vi "InitFPGA.vi"(2 "error in":errorcluster, 3 "FPGA VI In":refnum<k20>) -> (0 "error out":errorcluster, 1 "FPGA VI Reference Out":refnum<k20>)   [LabVIEW 2014]
doc: "Check for compatibility and Initilize FPGA."
uses:
  <vilib>/LabVIEW Targets/FPGA/FlexRIO/CustomFPGAMethods/79XXR_Method_IOModuleStatusImpl.vi
  <vilib>/Utility/error.llb/Error Cluster From Error Code.vi
  <vilib>/rvi/errors/niLvFpgaAdjustHostInterfaceError.vi
  <vilib>/rvi/interface/nirviMethod/nirviMethod.xnode
  <vilib>/rvi/interface/nirviReadWriteControl/nirviReadWriteControl.xnode
  NiFpgaLv.dll
  <vilib>/rvi/interface/Simulation/niFpgaSimulationCallBeginRW.vi
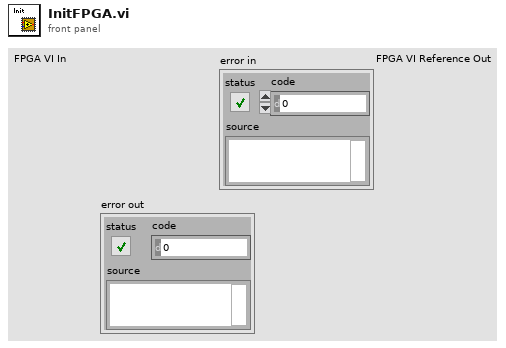
[diagram p1: front panel]
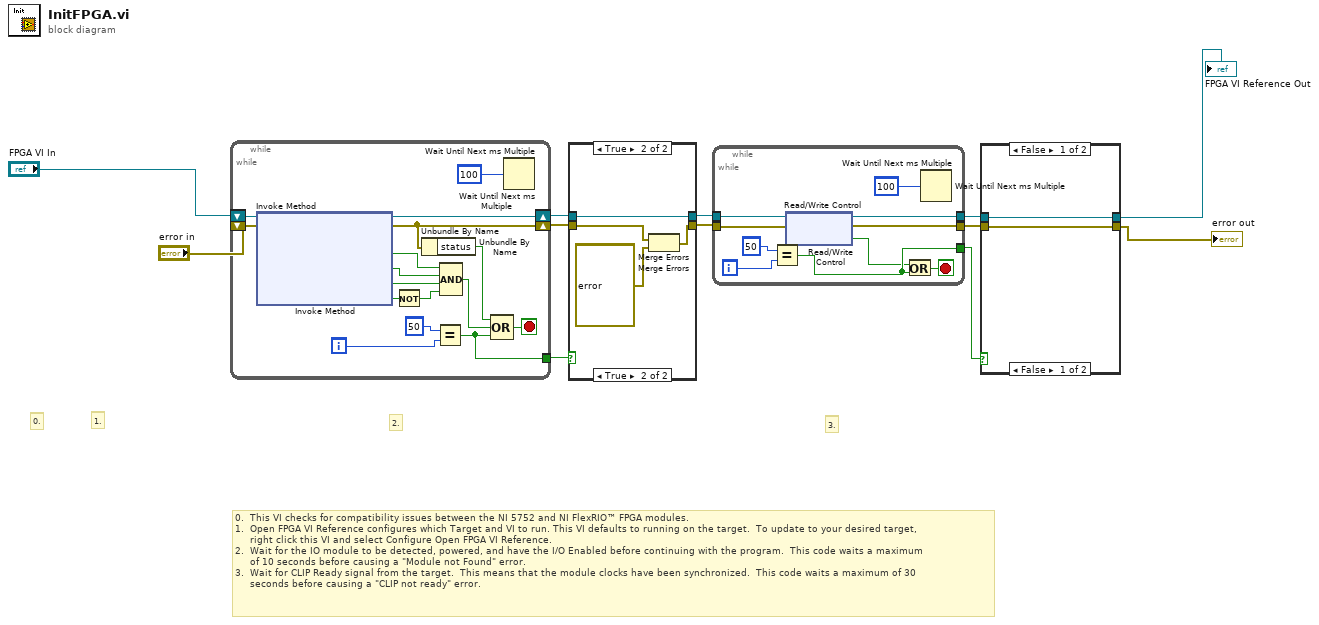
[diagram p0: block diagram]
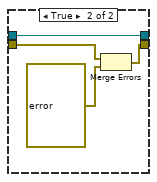
[diagram p2: hidden frame]
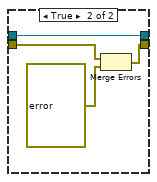
[diagram p4: hidden frame]
diagram:
  # "0.  This VI checks for compatibility issues between the NI 5752 and NI FlexRIO™ FPGA modules. \n1.  Open FPGA VI Reference configures which Target and VI to run. This VI defaults to running on the target.  To update to your desired target, \n     right click this VI and select Configure Open FPGA VI Reference.\n2.  Wait for the IO module to be detected, powered, and have the I/O Enabled before continuing with the program.  This code waits a maximum \n     of 10 seconds before causing a \"Module not Found\" error.\n3.  Wait for CLIP Ready signal from the target.  This means that the module clocks have been synchronized.  This code waits a maximum of 30 \n     seconds before causing a \"CLIP not ready\" error."
  # "0."
  # "3."
  # "1."
  # "0."
  # "3."
  # "2."
  # "1."
  n1 = while {
    shift-right: [w27] -> w20
    shift-left: "error in" -> [w35]
    shift-right: [w34] -> w18
    shift-left: "FPGA VI In" -> [w36]
    tunnel: [w23] -> w19
    i -> [w29]
    stop <- w24 stop-if-true
    n2 = xnode "Invoke Method"("FPGA VI Reference In"=w36, "error in"=w35) -> ("FPGA VI Reference Out"=w34:refnum<k20>, "error out"=w27:errorcluster, "IO Module Present?"=w33:bool, "Power Enabled?"=w32:bool, "IO Enabled?"=w31:bool, "IO Module Mismatch?"=w22:bool)
    n3 = Not(x=w22) -> (.not. x?=w21:bool)
    n4 = Unbundle By Name(w27) -> ("status"=w26:bool)
    n5 = Equal?(x=50, y=w29) -> (x = y?=w23:bool)
    n6 = Compound Arithmetic op=AND(w33, w32, w31, w21) -> (w25:bool)
    n7 = Compound Arithmetic op=OR(w26, w25, w23) -> (w24:bool)
    n8 = Wait Until Next ms Multiple(millisecond multiple=u32 100) -> ()  [unwired: 1 out]
  }
  n9 = while {
    shift-right: [w43] -> w4
    shift-left: _ -> [w51]
    shift-right: [w50] -> w6
    shift-left: _ -> [w52]
    tunnel: [w39] -> w5
    i -> [w45]
    stop <- w40 stop-if-true
    n10 = xnode "Invoke Method"("FPGA VI Reference In"=w52, "error in"=w51) -> ("FPGA VI Reference Out"=w50:refnum<k20>, "error out"=w43:errorcluster, "IO Module Present?"=w49:bool, "Power Enabled?"=w48:bool, "IO Enabled?"=w47:bool, "IO Module Mismatch?"=w38:bool)
    n11 = Not(x=w38) -> (.not. x?=w37:bool)
    n12 = Unbundle By Name(w43) -> ("status"=w42:bool)
    n13 = Equal?(x=50, y=w45) -> (x = y?=w39:bool)
    n14 = Compound Arithmetic op=AND(w49, w48, w47, w37) -> (w41:bool)
    n15 = Compound Arithmetic op=OR(w42, w41, w39) -> (w40:bool)
    n16 = Wait Until Next ms Multiple(millisecond multiple=u32 100) -> ()  [unwired: 1 out]
  }
  n17 = case shown="True" w19 {
    tunnel: w20 -> [w53 w57]
    tunnel: [w53 w56] -> w16
    tunnel: w18 -> [w54 w55]
    tunnel: [w54 w55] -> w17
    frame False {
    }
    frame True {
      n18 = Merge Errors(w57, errorcluster {"status"=TRUE, "code"=-1, "source"="The IO Module was not present, powered, or the IO were not enabled.  Verify the NI 5752 is securly connected and try again."} ("error in")) -> (w56:errorcluster)
    }
  }
  n19 = case shown="True" w5 {
    tunnel: w4 -> [w59 w63]
    tunnel: [w59 w62] -> w8
    tunnel: w6 -> [w60 w61]
    tunnel: [w60 w61] -> w7
    frame False {
    }
    frame True {
      n20 = Merge Errors(w63, errorcluster {"status"=TRUE, "code"=-1, "source"="The IO Module was not present, powered, or the IO were not enabled.  Verify the NI 5752 is securly connected and try again."} ("error in")) -> (w62:errorcluster)
    }
  }
  n21 = while {
    tunnel: w17 -> [w74]
    tunnel: [w70] -> w15
    tunnel: [w69] -> w14
    tunnel: [w67] -> w13
    tunnel: w16 -> [w65]
    i -> [w72]
    stop <- w68 stop-if-true
    n22 = Equal?(x=50, y=w72) -> (x = y?=w67:bool)
    n23 = xnode "Read/Write Control"("FPGA VI Reference In"=w74, "error in"=w65) -> ("FPGA VI Reference Out"=w70:refnum<k20>, "error out"=w69:errorcluster, "Init Done"=w66:bool)
    n24 = Or(x=w66, y=w67) -> (x .or. y?=w68:bool)
    n25 = Wait Until Next ms Multiple(millisecond multiple=u32 100) -> ()  [unwired: 1 out]
  }
  n26 = while {
    tunnel: w7 -> [w84]
    tunnel: [w80] -> w9
    tunnel: [w79] -> w10
    tunnel: [w77] -> w12
    tunnel: w8 -> [w75]
    i -> [w82]
    stop <- w78 stop-if-true
    n27 = Equal?(x=50, y=w82) -> (x = y?=w77:bool)
    n28 = xnode "Read/Write Control"("FPGA VI Reference In"=w84, "error in"=w75) -> ("FPGA VI Reference Out"=w80:refnum<k20>, "error out"=w79:errorcluster, "Init Done"=w76:bool)
    n29 = Or(x=w76, y=w77) -> (x .or. y?=w78:bool)
    n30 = Wait Until Next ms Multiple(millisecond multiple=u32 100) -> ()  [unwired: 1 out]
  }
  n31 = case shown="False" w13 {
    tunnel: w14 -> [w85 w89]
    tunnel: [w85 w88] -> _
    tunnel: w15 -> [w86 w87]
    tunnel: [w86 w87] -> _
    frame False {
    }
    frame True {
      n32 = Merge Errors(w89, errorcluster {"status"=TRUE, "code"=-1, "source"="The IO Module CLIP was not ready. If you are using any external clocks, make sure they are connected and within the supported specifications."} ("error in")) -> (w88:errorcluster)
    }
  }
  n33 = case shown="False" w12 {
    tunnel: w10 -> [w91 w95]
    tunnel: [w91 w94] -> w11
    tunnel: w9 -> [w92 w93]
    tunnel: [w92 w93] -> w3
    frame False {
    }
    frame True {
      n34 = Merge Errors(w95, errorcluster {"status"=TRUE, "code"=-1, "source"="The IO Module CLIP was not ready. If you are using any external clocks, make sure they are connected and within the supported specifications."} ("error in")) -> (w94:errorcluster)
    }
  }
  "error out" <- w11
  "FPGA VI Reference Out" <- w3
